vi "assign FPGA resources.vi"(8 "error in (no error)":errorcluster, 11 "Device Item Ref in":T1 format="%.0x") -> (0 "error out":errorcluster, 2 "Variant":variant, 3 "Device Item Ref out":T1 format="%.0x")   [LabVIEW 2016, in "FPGA Addon System Explorer.lvlib"]
uses:
  FPGA Addon System Explorer.lvlib
  <vilib>/NI Veristand/Custom Device API/Custom Device Item Ref.ctl
  Shared/Constants.vi
  <vilib>/NI Veristand/Custom Device API/Get Item Property (String).vi
  <vilib>/NI Veristand/Custom Device API/Get Item Property (Variant).vi
  <vilib>/NI Veristand/Custom Device API/Set Item Property (Variant).vi
  RM Client API/FPGA RM Client API.lvlib
  <vilib>/NI VeriStand/Custom Device API/Custom Device API.lvlib
  Shared/FPGA Addon Shared.lvlib
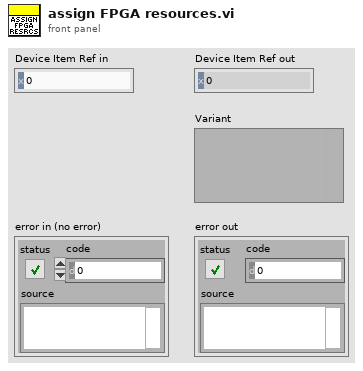
[diagram p1: front panel]
types:
  T1 = typedef "Custom Device API.lvlib/Custom Device Item Ref.ctl" = u64
  T2 = typedef "FPGA RM Client API.lvlib/fpga resource.ctl" = cluster{"name":string, "datatype":string, "channel type":T3, "value":variant, "notes":string}
  T3 = typedef "FPGA RM Client API.lvlib/Channel Type.ctl" = enum16{"Write Channel", "Read Channel", "Write Waveform", "Read Waveform"}
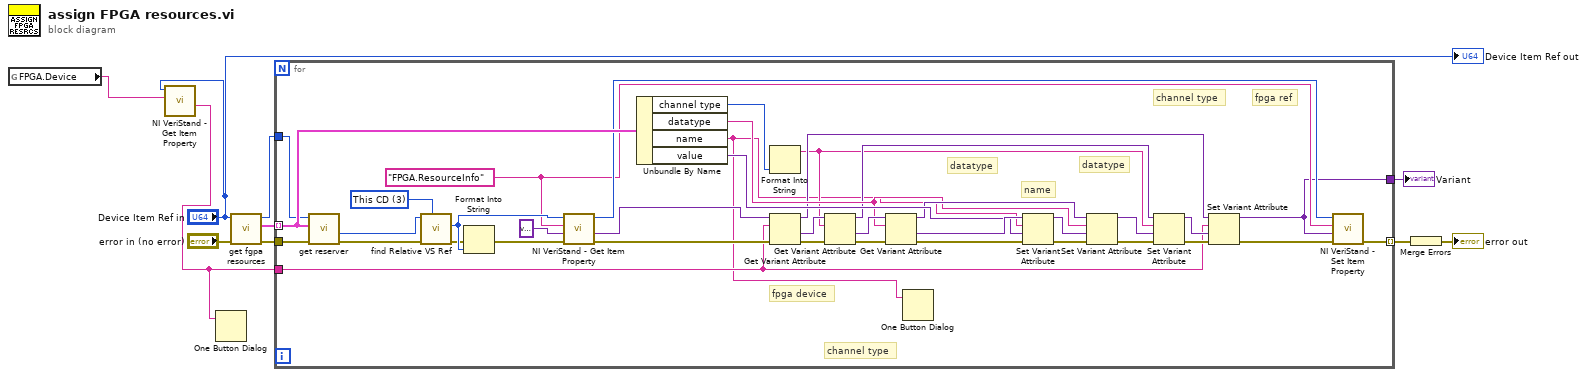
[diagram p0: block diagram]
diagram:
  n1 = global read "Constants.vi" "FPGA.Device"() -> (w3:string)
  n2 = call-poly <vilib>:"NI VeriStand - Get Item Property.vi"("Property Name"=w3, "Item Ref in"="Device Item Ref in") -> ("Value"=w1:string)  [unwired: 6 in, 3 out]
  n3 = One Button Dialog(message=w1) -> ()  [unwired: 1 in, 1 out]
  n4 = call "get fgpa resources.vi"("error in (no error)"="error in (no error)", "Item Ref in"="Device Item Ref in") -> ("error out"=w10:errorcluster, "get fpga resources"=w7:T2[], "Item Ref out"=w8:T1)  [unwired: 6 in, 1 out]
  n5 = for {
    tunnel: w7 -> [w46] mode=indexing
    tunnel: w8 -> [w15]
    tunnel: w10 -> [w35]
    tunnel: [w21] -> w6 mode=indexing
    tunnel: [w13] -> w4
    tunnel: w1 -> [w12]
    w23 = "FPGA.ResourceInfo" ("Property Name")
    w28 = u16 3 items=["Targets", "Controller", "Custom Devices", "This CD", "This CD/Group", "This CD/Group/SubGroup"] ("Relative Type")
    # "fpga ref"
    # "channel type"
    # "datatype"
    # "name"
    # "datatype"
    # "channel type"
    # "fpga device"
    n6 = call "get reserver.vi"("error in (no error)"=w35, "FPGA Resource"=w46, "Item Ref in"=w15) -> ("error out"=w20:errorcluster, "Dependent Node Ref"=w29:T1)  [unwired: 5 in, 2 out]
    n7 = call "find Relative VS Ref.vi"("Relative Type"=w28, "error in (no error)"=w20, "Item Ref in"=w29) -> ("error out"=w19:errorcluster, "Relative Item Ref Out"=w27:T1)  [unwired: 4 in, 3 out]
    n8 = Format Into String(error in=w19, w27) -> (error out=w18:errorcluster)  [unwired: 2 in, 1 out]
    n9 = call-poly <vilib>:"NI VeriStand - Get Item Property.vi"("error in (no error)"=w18, "Default Value"=variant, "Property Name"=w23, "Item Ref in"=w27) -> ("error out"=w14:errorcluster, "Value"=w25:variant, "Item Ref out"=w24:T1)  [unwired: 4 in, 1 out]
    n10 = Unbundle By Name(w46) -> ("channel type"=w17:T3, "datatype"=w41:string, "name"=w11:string, "value"=w44:variant)
    n11 = Format Into String(w17) -> (resulting string=w16:string)  [unwired: 3 in, 1 out]
    n12 = Get Variant Attribute(Variant=w25, name=w12, error in=w14) -> (duplicate Variant=w36:variant, value=w48:variant, error out=w34:errorcluster)  [unwired: 1 in, 1 out]
    n13 = Get Variant Attribute(Variant=w48, name=w16, error in=w34) -> (duplicate Variant=w39:variant, value=w47:variant, error out=w33:errorcluster)  [unwired: 1 in, 1 out]
    n14 = Get Variant Attribute(Variant=w47, name=w41, error in=w33) -> (duplicate Variant=w42:variant, value=w45:variant, error out=w32:errorcluster)  [unwired: 1 in, 1 out]
    n15 = One Button Dialog(message=w11) -> ()  [unwired: 1 in, 1 out]
    n16 = Set Variant Attribute(Variant=w45, name=w11, value=w44, error in=w32) -> (Variant out=w43:variant, error out=w31:errorcluster)  [unwired: 1 out]
    n17 = Set Variant Attribute(Variant=w42, name=w41, value=w43, error in=w31) -> (Variant out=w40:variant, error out=w30:errorcluster)  [unwired: 1 out]
    n18 = Set Variant Attribute(Variant=w39, name=w16, value=w40, error in=w30) -> (Variant out=w37:variant, error out=w38:errorcluster)  [unwired: 1 out]
    n19 = Set Variant Attribute(Variant=w36, name=w12, value=w37, error in=w38) -> (Variant out=w13:variant, error out=w22:errorcluster)  [unwired: 1 out]
    n20 = call-poly <vilib>:"NI VeriStand - Set Item Property.vi"("error in (no error)"=w22, "Value"=w13, "Property Name"=w23, "Item Ref in"=w24) -> ("error out"=w21:errorcluster)  [unwired: 5 in, 2 out]
  }
  "Variant" <- w4
  n21 = Merge Errors(w6) -> (→"error out":errorcluster)
  "Device Item Ref out" <- "Device Item Ref in"
